vi "VrmVISAFindInsrument.vi"() -> (0 "error out":errorcluster, 2 "Cancelled":bool, 3 "VISA resource name out":refnum<visa-resource-name>)   [LabVIEW 2011]
panel:
  in  "Port":i32=33575
  in  "IP address":string="127.0.0.1"
  in  "Cancel":bool
  in  "OK":bool
  out "Result":string
  in  "Test":bool
  # "1. Select IP address\n2. Select port number\n3. Test the connection\n4. If successful, click on OK"
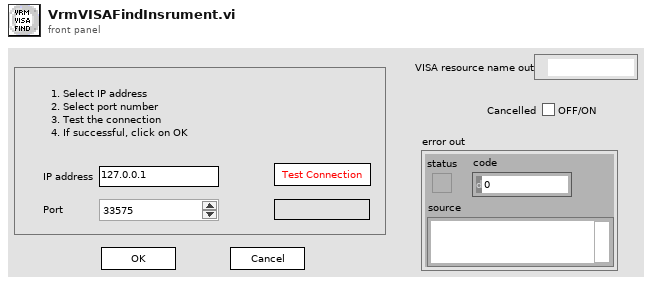
[diagram p1: front panel]
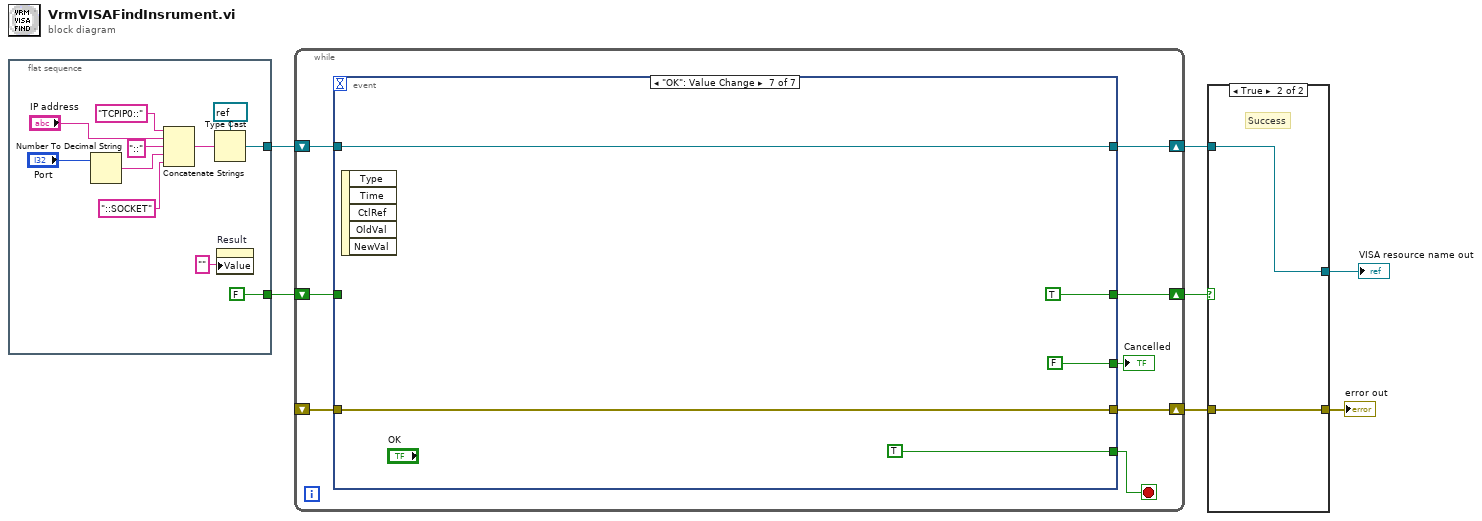
[diagram p0: block diagram]
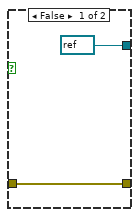
[diagram p2: hidden frame]
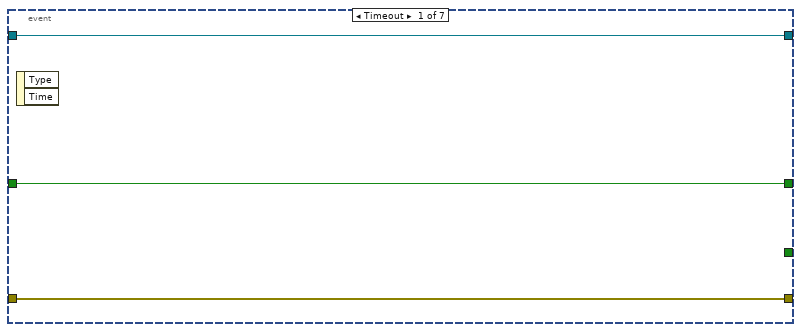
[diagram p3: hidden frame]
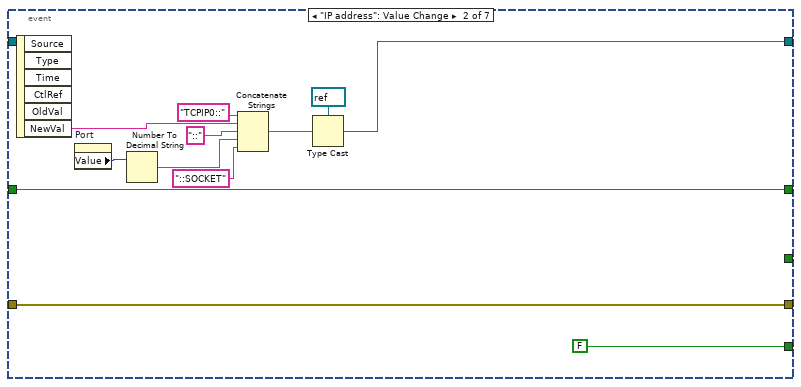
[diagram p4: hidden frame]
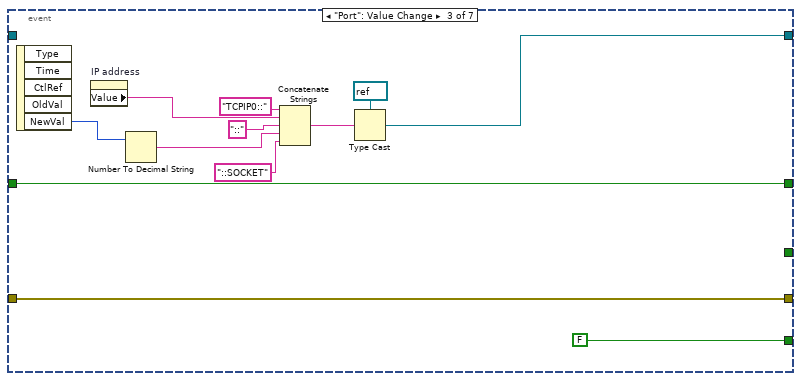
[diagram p5: hidden frame]
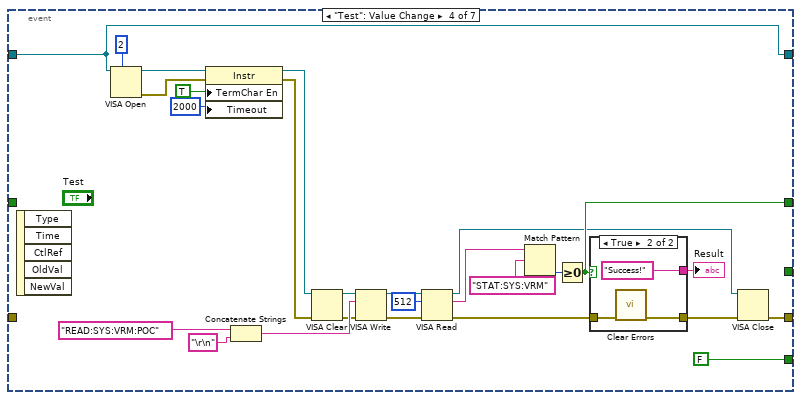
[diagram p6: hidden frame]
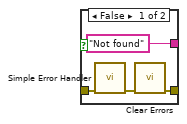
[diagram p7: hidden frame]
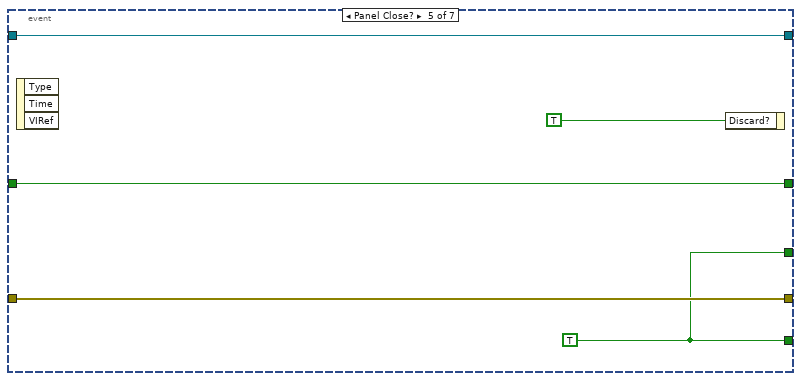
[diagram p8: hidden frame]
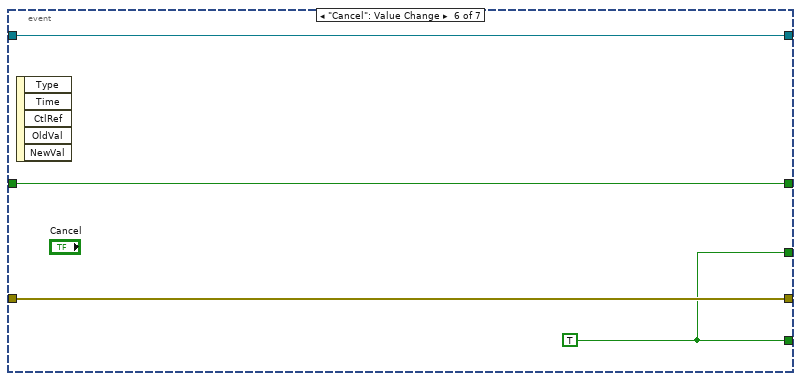
[diagram p9: hidden frame]
diagram:
  n1 = flat-sequence {
    tunnel: [w9] -> w2
    tunnel: [FALSE] -> w1
    frame #0 {
      n2 = Number To Decimal String(number="Port") -> (decimal integer string=w12:string)  [unwired: 1 in]
      n3 = Concatenate Strings("TCPIP0::" ("string"), "IP address", "::" ("string"), w12, "::SOCKET" ("string")) -> (w10:string)
      n4 = Type Cast(type=refnum<visa-resource-name> refnum ("VISA resource name"), x=w10) -> (*(type *) &x=w9:refnum<visa-resource-name>)
      n5 = property on="Result" class="Str"("Value"="" ("Result")) -> ()  [unwired: 2 in, 2 out]
    }
  }
  n6 = while {
    shift-right: [w25] -> w7
    shift-left: w1 -> [w24]
    shift-right: [w23] -> w6
    shift-left: w2 -> [w22]
    shift-right: [w21] -> w5
    shift-left: _ -> [w20]
    stop <- w26 stop-if-true
    n7 = event shown="[6] \"OK\": Value Change" {
      selector: _ -> [_ _ _ _ _ _ _]
      dyn-events: _ -> [_ _ _ _ _ _ _]
      timeout: _ -> [_ _ _ _ _ _ _]
      tunnel: [_ FALSE FALSE FALSE w87 w92 TRUE] -> w26
      tunnel: [w27 w39 w51 w65 w89 w93 w98] -> w21
      tunnel: [w29 w40 w52 w68 w91 w95 TRUE] -> w25
      tunnel: w24 -> [w29 w40 w52 _ w91 w95 _]
      tunnel: [w28 w30 w44 w54 w90 w94 w99] -> w23
      tunnel: w22 -> [w28 _ _ w54 w90 w94 w99]
      tunnel: w20 -> [w27 w39 w51 _ w89 w93 w98]
      tunnel: [_ _ _ _ w87 w92 FALSE ("Discard?")] -> w19
      event Timeout {
        n8 = event-data() -> ()  [unwired: 1 in, 2 out]
      }
      event "IP address": Value Change {
        n9 = event-data() -> ("NewVal"=w31:string)  [unwired: 1 in, 5 out]
        n10 = property on="Port" class="DigNum (strict)"() -> ("Value"=w32:i32)  [unwired: 2 in, 2 out]
        n11 = Number To Decimal String(number=w32) -> (decimal integer string=w35:string)  [unwired: 1 in]
        n12 = Concatenate Strings("TCPIP0::" ("string"), w31, "::" ("string"), w35, "::SOCKET" ("string")) -> (w33:string)
        n13 = Type Cast(type=refnum<visa-resource-name> refnum ("VISA resource name"), x=w33) -> (*(type *) &x=w30:refnum<visa-resource-name>)
      }
      event "Port": Value Change {
        n14 = event-data() -> ("NewVal"=w43:i32)  [unwired: 1 in, 4 out]
        n15 = property on="IP address" class="Str"() -> ("Value"=w42:string)  [unwired: 2 in, 2 out]
        n16 = Number To Decimal String(number=w43) -> (decimal integer string=w47:string)  [unwired: 1 in]
        n17 = Concatenate Strings("TCPIP0::" ("string"), w42, "::" ("string"), w47, "::SOCKET" ("string")) -> (w45:string)
        n18 = Type Cast(type=refnum<visa-resource-name> refnum ("VISA resource name"), x=w45) -> (*(type *) &x=w44:refnum<visa-resource-name>)
      }
      event "Test": Value Change {
        n19 = event-data() -> ()  [unwired: 1 in, 5 out]
        n20 = VISA Open(timeout (0)=u32 2 ("VISA Open timeout (0)"), VISA resource name=w54) -> (VISA resource name=w57:refnum<visa-resource-name>, error out=w56:errorcluster)  [unwired: 3 in]
        n21 = property class="Instr"(reference=w57, error in=w56, "TermChar En"=TRUE ("Message Based Settings:Termination Character Enable"), "Timeout"=u32 2000 ("General Settings:Timeout Value")) -> (reference out=w61:refnum<visa-resource-name>, error out=w60:errorcluster)
        n22 = Concatenate Strings("READ:SYS:VRM:POC" ("Command to send"), "\r\n") -> (w76:string)
        n23 = VISA Clear(VISA resource name=w61, error in (no error)=w60) -> (VISA resource name out=w62:refnum<visa-resource-name>, error out=w59:errorcluster)
        n24 = VISA Write(VISA resource name=w62, write buffer=w76, error in (no error)=w59) -> (VISA resource name out=w78:refnum<visa-resource-name>, error out=w79:errorcluster)  [unwired: 1 out]
        n25 = VISA Read(VISA resource name=w78, byte count=u32 512, error in (no error)=w79) -> (VISA resource name out=w64:refnum<visa-resource-name>, read buffer=w72:string, error out=w69:errorcluster)  [unwired: 1 out]
        n26 = Match Pattern(string=w72, regular expression="STAT:SYS:VRM") -> (offset past match=w71:i32)  [unwired: 1 in, 3 out]
        n27 = Greater Or Equal To 0?(x=w71) -> (x >= 0?=w68:bool)
        n28 = case shown="True" w68 {
          tunnel: ["Not found" ("read buffer") "Success!" ("read buffer")] -> w70
          tunnel: w69 -> [w83 w85]
          tunnel: [w81 w84] -> w63
          frame False {
            n29 = call <vilib>:"Simple Error Handler.vi"("error in (no error)"=w83) -> ("error out"=w80:errorcluster)  [unwired: 4 in, 4 out]
            n30 = call <vilib>:"Clear Errors.vi"("error in (no error)"=w80) -> ("error out"=w81:errorcluster)  [unwired: 6 in]
          }
          frame True {
            n31 = call <vilib>:"Clear Errors.vi"("error in (no error)"=w85) -> ("error out"=w84:errorcluster)  [unwired: 6 in]
          }
        }
        "Result" <- w70
        n32 = VISA Close(VISA resource name=w64, error in (no error)=w63) -> (error out=w65:errorcluster)
      }
      event Panel Close? {
        w87 = TRUE
        n33 = event-data() -> ()  [unwired: 1 in, 3 out]
        n34 = event-data("Discard?"=TRUE) -> ()  [unwired: 1 in, 1 out]
      }
      event "Cancel": Value Change {
        w92 = TRUE
        n35 = event-data() -> ()  [unwired: 1 in, 5 out]
      }
      event "OK": Value Change {
        n36 = event-data() -> ()  [unwired: 1 in, 5 out]
      }
    }
    "Cancelled" <- w19
  }
  n37 = case shown="True" w7 {
    tunnel: w6 -> [_ w103]
    tunnel: w5 -> [w102 w104]
    tunnel: [w102 w104] -> w4
    tunnel: [refnum<visa-resource-name> refnum ("VISA resource name out") w103] -> w3
    frame False {
    }
    frame True {
      # "Success"
    }
  }
  "error out" <- w4
  "VISA resource name out" <- w3
